vi "REQ Initialize Hardware.vi"(6 "wait for reply (T)":bool=TRUE, 8 "error in":errorcluster, 11 "Connection Setting":T1) -> (0 "error out":errorcluster, 1 "timed out?":bool, 3 "Connect?":bool)   [LabVIEW 2016, in "DC PWS.lvlib"]
doc: "_____\nCreated using DQMH Event Scripter 6.1.0.128."
uses:
  DC PWS.lvlib
  REQ Initialize Hardware Argument--cluster.ctl
  REQ Initialize Hardware (Reply Payload)--cluster.ctl
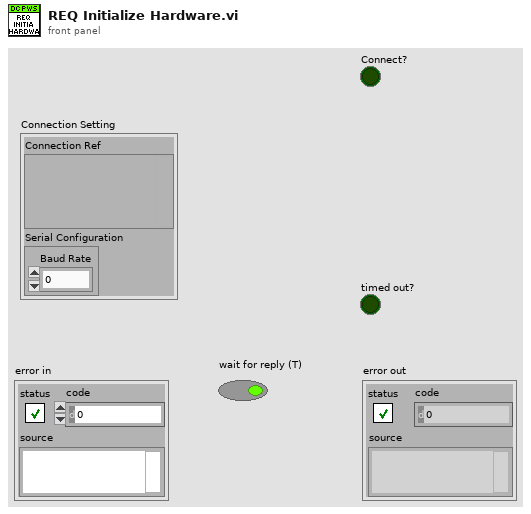
[diagram p1: front panel]
types:
  T1 = cluster{"Connection Ref":variant, "Serial Configuration":cluster{"Baud Rate":u32}}
  T2 = typedef "DC PWS.lvlib/REQ Initialize Hardware Argument--cluster.ctl" = cluster{"Connection Setting":cluster{"Connection Ref":variant, "Serial Configuration":cluster{"Baud Rate":u32}}, "Wait Notifier":refnum<notifier>, "wait for reply":bool}
  T3 = typedef "DC PWS.lvlib/Request Events--cluster.ctl" = cluster{"Stop Module":refnum<user-event>, "Show Panel":refnum<user-event>, "Hide Panel":refnum<user-event>, "Get Module Execution Status":refnum<user-event>, "Show Diagram":refnum<user-event>, "REQ Initialize Hardware":refnum<user-event>, "REQ Config Current Limit":refnum<user-event>, "REQ Over Voltage Limit":refnum<user-event>, "REQ Configure Output":refnum<user-event>, "REQ Enable Output":refnum<user-event>, "REQ Measurement":refnum<user-event>, "REQ Close Ref":refnum<user-event>}
  T4 = typedef "DC PWS.lvlib/REQ Initialize Hardware (Reply Payload)--cluster.ctl" = cluster{"Connect?":bool, "error":errorcluster}
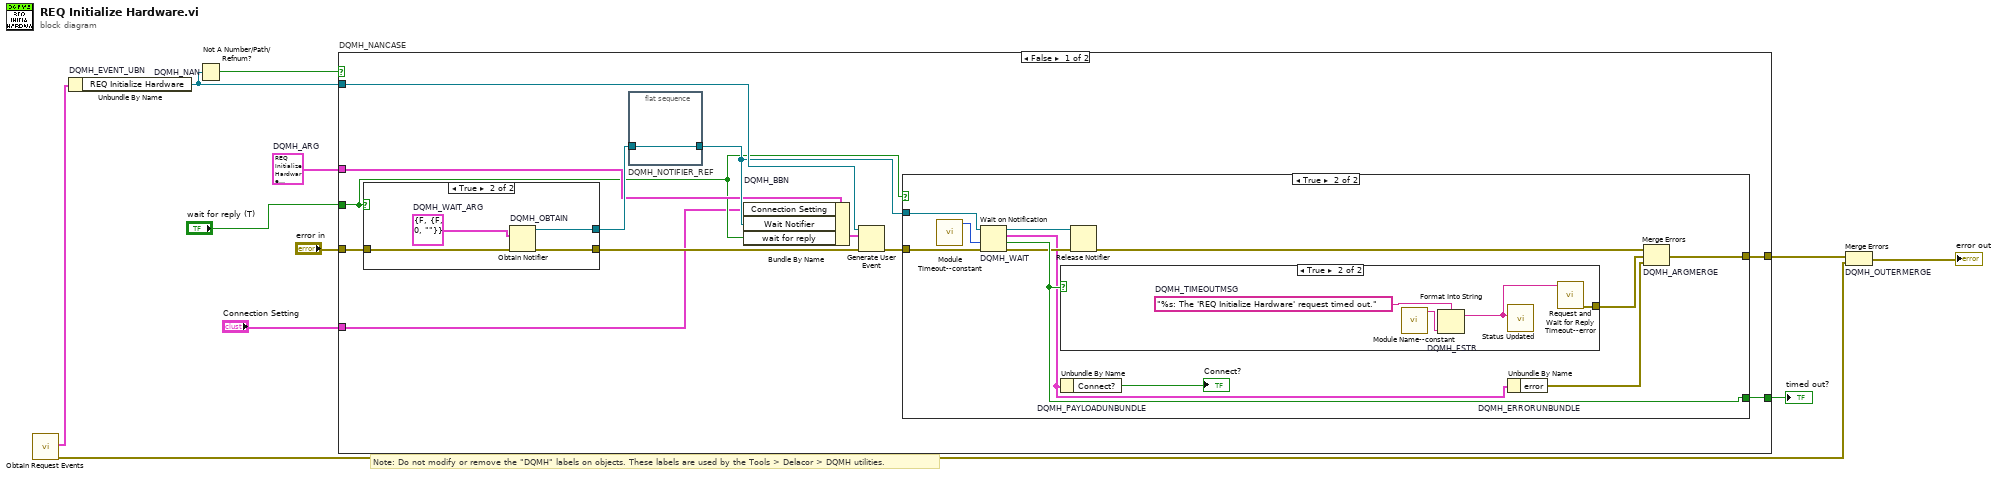
[diagram p0: block diagram]
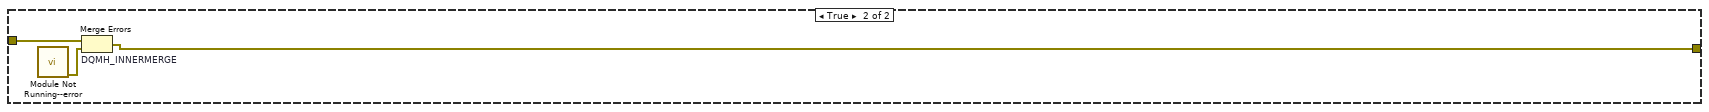
[diagram p5: hidden frame]
diagram:
  w5 = T2 {"Connection Setting"={"Connection Ref"=variant, "Serial Configuration"={"Baud Rate"=9600}}, "Wait Notifier"=refnum, "wait for reply"=FALSE}  # DQMH_ARG
  # "Note: Do not modify or remove the \"DQMH\" labels on objects. These labels are used by the Tools > Delacor > DQMH utilities."
  n1 = call "Obtain Request Events.vi"() -> ("error out"=w3:errorcluster, "DC PWS Request Events"=w2:T3)  [unwired: 10 in]
  n2 = Unbundle By Name "DQMH_EVENT_UBN"(w2) -> ("REQ Initialize Hardware"=w9:refnum<user-event>)
  n3 = Not A Number/Path/Refnum? "DQMH_NAN"(number/path/refnum=w9) -> (NaN/Path/Refnum?=w8:bool)
  n4 = case "DQMH_NANCASE" shown="False" w8 {
    tunnel: "error in" -> [w23 w49]
    tunnel: w9 -> [w21 _]
    tunnel: [w18 w48] -> w6
    tunnel: [w19 _] -> w7
    tunnel: w5 -> [w14 _]
    tunnel: "wait for reply (T)" -> [w13 _]
    tunnel: "Connection Setting" -> [w12 _]
    frame False {
      n5 = case shown="True" w13 {
        tunnel: w23 -> [w42 w46]
        tunnel: [w42 w45] -> w20
        tunnel: [_ w43] -> w16
        frame False {
        }
        frame True {
          w44 = T4 {"Connect?"=FALSE, "error"={"status"=FALSE, "code"=0, "source"=""}}  # DQMH_WAIT_ARG
          n6 = Obtain Notifier "DQMH_OBTAIN"(notification data type=w44, error in (no error)=w46) -> (notifier out=w43:refnum<notifier>, error out=w45:errorcluster)  [unwired: 2 in, 1 out]
        }
      }
      n7 = flat-sequence "DQMH_NOTIFIER_REF" {
        tunnel: w16 -> [w24]
        tunnel: [w24] -> w15
        frame #0 {
        }
      }
      n8 = Bundle By Name "DQMH_BBN"(cluster=w14, "Connection Setting"=w12, "Wait Notifier"=w15, "wait for reply"=w13) -> (w17:T2)
      n9 = Generate User Event(user event=w21, event data cluster=w17, error in=w20) -> (error out=w22:errorcluster)  [unwired: 1 in, 1 out]
      n10 = case shown="True" w13 {
        tunnel: w22 -> [w25 w37]
        tunnel: w15 -> [_ w36]
        tunnel: [_ w34] -> w19
        tunnel: [w25 w33] -> w18
        frame False {
        }
        frame True {
          n11 = call "Module Timeout--constant.vi"() -> ("Module Timeout"=w27:i32)  [unwired: 11 in]
          n12 = Wait on Notification "DQMH_WAIT"(notifier=w36, timeout in ms (-1)=w27, error in (no error)=w37) -> (notifier out=w35:refnum<notifier>, notification=w28:T4, timed out?=w34:bool, error out=w32:errorcluster)  [unwired: 1 in]
          n13 = case shown="True" w34 {
            tunnel: [_ w39] -> w29
            frame False {
            }
            frame True {
              w41 = "%s: The 'REQ Initialize Hardware' request timed out."  # DQMH_TIMEOUTMSG
              n14 = call "Module Name--constant.vi"() -> ("Module Name"=w38:string)  [unwired: 11 in]
              n15 = Format Into String "DQMH_FSTR"(format string=w41, w38) -> (resulting string=w40:string)  [unwired: 2 in, 1 out]
              n16 = call "Status Updated.vi"("Status"=w40) -> ()  [unwired: 10 in, 1 out]
              n17 = call "Request and Wait for Reply Timeout--error.vi"("Error Message"=w40) -> ("error out"=w39:errorcluster)  [unwired: 10 in]
            }
          }
          n18 = Unbundle By Name "DQMH_PAYLOADUNBUNDLE"(w28) -> ("Connect?"=→"Connect?":bool)
          n19 = Release Notifier(notifier=w35, error in (no error)=w32) -> (error out=w31:errorcluster)  [unwired: 1 in, 2 out]
          n20 = Unbundle By Name "DQMH_ERRORUNBUNDLE"(w28) -> ("error"=w30:errorcluster)
          n21 = Merge Errors "DQMH_ARGMERGE"(w31, w29, w30) -> (w33:errorcluster)
        }
      }
    }
    frame True {
      n22 = call "Module Not Running--error.vi"() -> ("error out"=w47:errorcluster)  [unwired: 11 in]
      n23 = Merge Errors "DQMH_INNERMERGE"(w49, w47) -> (w48:errorcluster)
    }
  }
  "timed out?" <- w7
  n24 = Merge Errors "DQMH_OUTERMERGE"(w6, w3) -> (→"error out":errorcluster)
